vi "Square Root - CM.vi"(1 "Complex Matrix A":T1) -> (0 "sqrt(A)":T1)   [LabVIEW 2020, in "NI_Matrix.lvlib"]
doc: "Computes the square root of the input matrix."
uses:
  NI_Matrix.lvlib
  ComplexMatrix.ctl
  NI_AALBase.lvlib
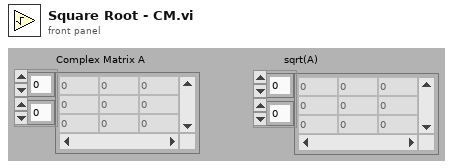
[diagram p1: front panel]
types:
  T1 = typedef "NI_Matrix.lvlib/ComplexMatrix.ctl" = cdb[][]
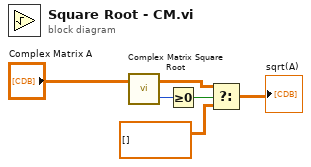
[diagram p0: block diagram]
diagram:
  n1 = call "Complex Matrix Square Root.vi"("Input Matrix"="Complex Matrix A") -> ("error"=w1:i32, "Matrix Square Root"=w2:T1)  [unwired: 1 in]
  n2 = Greater Or Equal To 0?(x=w1) -> (x >= 0?=w6:bool)
  n3 = Select(t=w2, s=w6, f=T1 [] ("A + B")) -> (s? t:f=→"sqrt(A)":T1)
